vi "mousePlusKeyboard.vi"() -> ()   [LabVIEW 2019]
uses:
  <vilib>/Utility/inputDevices.llb/keyboardAcquire.vi
  <vilib>/Utility/inputDevices.llb/mouseAcquire.vi
  <vilib>/Utility/inputDevices.llb/closeKeyboard.vi
  <vilib>/Utility/inputDevices.llb/closeMouse.vi
panel:
  out "keys pressed":T1(array[ring])
  out "clava":errorcluster
  out "number":u32
  out "array":bool[](array[boolean])
  out "Waveform Chart":T2(graph)
  in  "stop":bool
  out "button info":T3
  out "axis info":T2
  in  "key mode":enum16{"RELATIVE", "ABSOLUTE"}(ring)=enum."ABSOLUTE"
  out "mouse":errorcluster
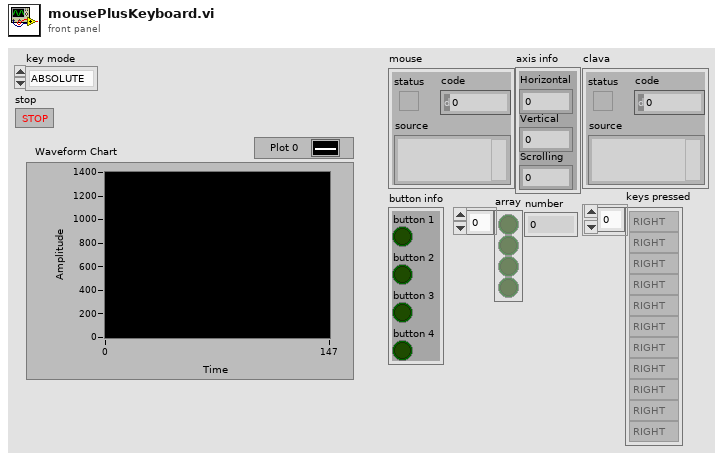
[diagram p1: front panel]
types:
  T1 = enum16{"0", "1", "2", "3", "4", "5", "6", "7", "8", "9", "A", "B", "C", "D", "E", "F", "G", "H", "I", "J", "K", "L", "M", "N", "O", "P", "Q", "R", "S", "T", "U", "V", "W", "X", "Y", "Z", "F1", "F2", "F3", "F4", "F5", "F6", "F7", "F8", "F9", "F10", "F11", "F12", "F13", "F14", "F15", "ADD", "BACK", "BACKSLASH", "CAPITAL", "COMMA", "DECIMAL", "DELETE", "DIVIDE", "DOWN", "END", "EQUALS", "ESCAPE", "GRAVE (`)", "HOME", "INSERT", "LBRACKET", "LCONTROL", "LEFT", "L ALT", "LSHIFT", "LWIN", "MINUS", "MULTIPLY", "NEXT", "NUMLOCK", "NUMPAD_0", "NUMPAD_1", "NUMPAD_2", "NUMPAD_3", "NUMPAD_4", "NUMPAD_5", "NUMPAD_6", "NUMPAD_7", "NUMPAD_8", "NUMPAD_9", "PAUSE", "PERIOD", "PRIOR (PG UP)", "RBRACKET", "RCONTROL", "RETURN", "RIGHT", "R ALT", "RSHIFT", "RWIN", "SCROLL", "SEMICOLON", "SLASH", "SPACE", "SUBTRACT", "TAB", "UP", "ENTER (num pad)", "' (quote)"}[]
  T2 = cluster{"Horizontal":i32, "Vertical":i32, "Scrolling":i32}
  T3 = cluster{"button 1":bool, "button 2":bool, "button 3":bool, "button 4":bool}
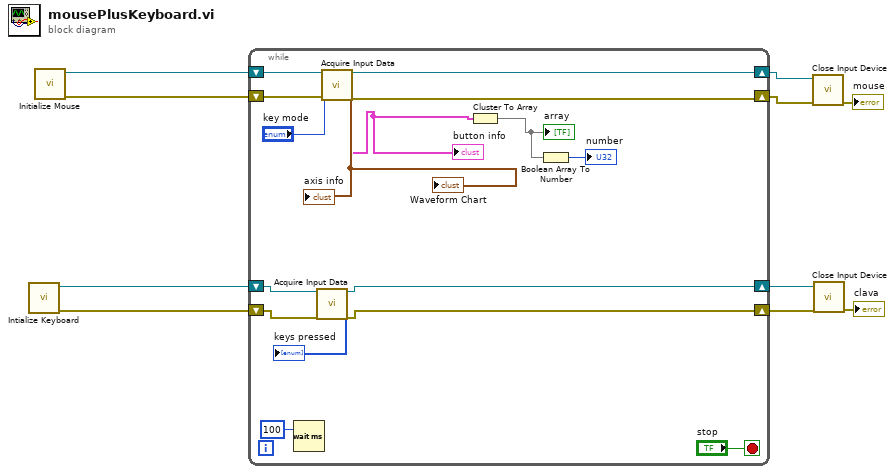
[diagram p0: block diagram]
diagram:
  n1 = call <vilib>:"Intialize Keyboard.vi"() -> ("error out"=w4:errorcluster, "device ID"=w5:refnum<k1>)  [unwired: 10 in]
  n2 = call <vilib>:"Initialize Mouse.vi"() -> ("error out"=w9:errorcluster, "device ID"=w10:refnum<k1>)  [unwired: 10 in]
  n3 = while {
    shift-right: [w24] -> w8
    shift-left: w10 -> [w26]
    shift-right: [w23] -> w7
    shift-left: w9 -> [w25]
    shift-right: [w13] -> w3
    shift-left: w5 -> [w15]
    shift-right: [w12] -> w2
    shift-left: w4 -> [w14]
    stop <- "stop" stop-if-true
    n4 = Wait (ms)(milliseconds to wait=u32 100) -> ()  [unwired: 1 out]
    n5 = call-poly <vilib>:"Acquire Input Data.vi"("device ID"=w15, "error in (no error)"=w14) -> ("device ID"=w13:refnum<k1>, "keys pressed"=→"keys pressed":T1, "error out"=w12:errorcluster)  [unwired: 15 in]
    n6 = call-poly <vilib>:"Acquire Input Data.vi"("device ID"=w26, "key mode"="key mode", "error in (no error)"=w25) -> ("device ID"=w24:refnum<k1>, "axis info"=→"axis info" →"Waveform Chart":T2, "button info"=w18:T3, "error out"=w23:errorcluster)  [unwired: 13 in]
    "button info" <- w18
    n7 = Cluster To Array(cluster=w18) -> (array=w17:bool[])
    "array" <- w17
    n8 = Boolean Array To Number(Boolean array=w17) -> (number=→"number":u32)
  }
  n9 = call-poly <vilib>:"Close Input Device.vi"("error in (no error)"=w7, "device ID"=w8) -> ("error out"=→"mouse":errorcluster)  [unwired: 8 in]
  n10 = call-poly <vilib>:"Close Input Device.vi"("error in (no error)"=w2, "device ID"=w3) -> ("error out"=→"clava":errorcluster)  [unwired: 8 in]
